vi "Main.vi"() -> ()   [LabVIEW 2019]
uses:
  controls/Data.ctl
  controls/UIRef.ctl
  controls/daqtypedef.ctl
  <vilib>/measure/NI_MABase.lvlib
panel:
  in  "Acquire":bool
  in  "Exit":bool
  out "Raw Data":waveform(dbl)(graph)
  out "Status Bar":string
  # "Laboratorium OSP"
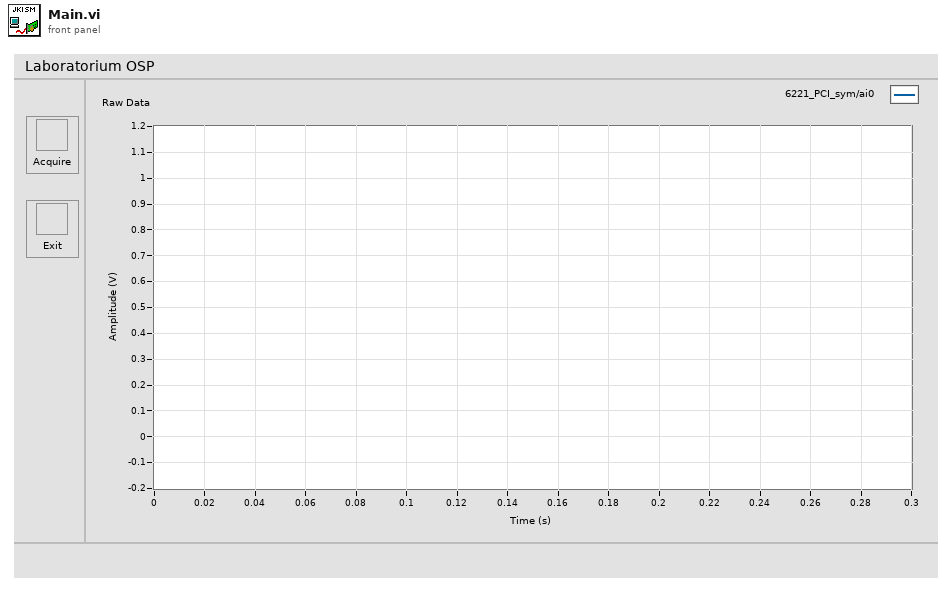
[diagram p1: front panel]
types:
  T1 = enum32{"Invalid", "Standard", "Closed", "Hidden", "Minimized", "Maximized"}
  T2 = enum32{"invalid app kind", "Development System", "Run Time System", "Student Edition", "Embedded LabVIEW", "Evaluation", "Custom"}
  T3 = typedef "Data.ctl" = cluster{"UICtlRef":T4, "DAQmxChannel":T5, "DAQmx Task Name":refnum<k21>, "Acquired Signal":waveform(dbl), "configuration file path":path, "taskout":refnum<k21>}
  T4 = typedef "UIRef.ctl" = cluster{"Acquire Btn":refnum<vi>, "Exit Btn":refnum<vi>, "Status":refnum<vi>, "WGraph":refnum<vi>}
  T5 = typedef "daqtypedef.ctl" = cluster{"PhysicalChanName":tag, "AI.Max":dbl, "AI.Min":dbl, "SampQuant.SampPerChan":dbl, "SampClk.Rate":dbl}
  T6 = cluster{"Core":cluster{"Current VI Reference":refnum<vi>, "Close Panel on Exit?":bool}, "Data":T3}
  T7 = cluster{"Current VI Reference":refnum<vi>, "Close Panel on Exit?":bool}
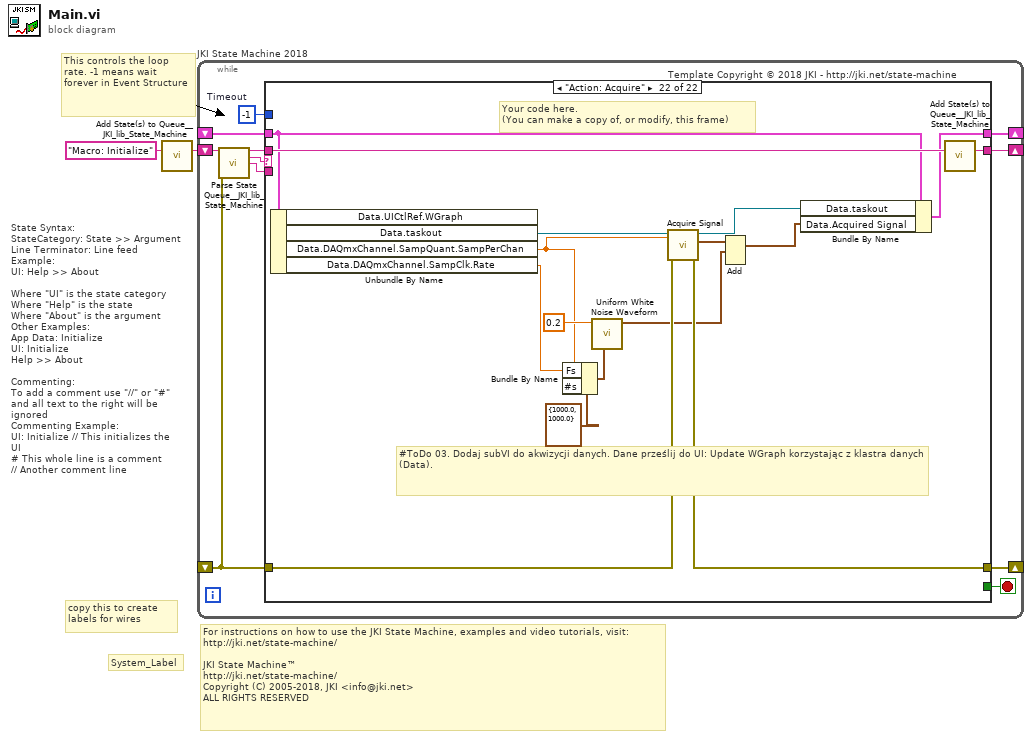
[diagram p0: block diagram]
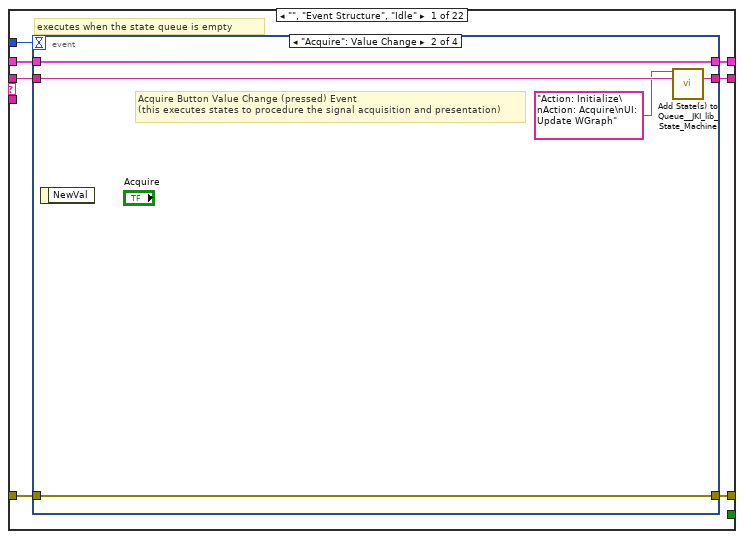
[diagram p2: hidden frame]
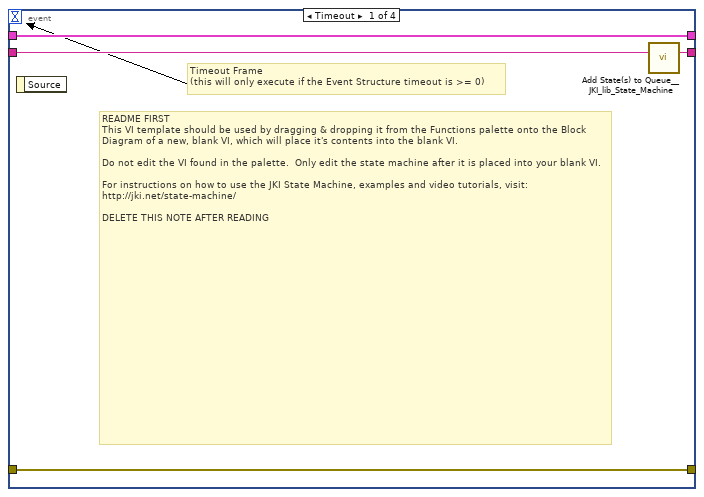
[diagram p3: hidden frame]
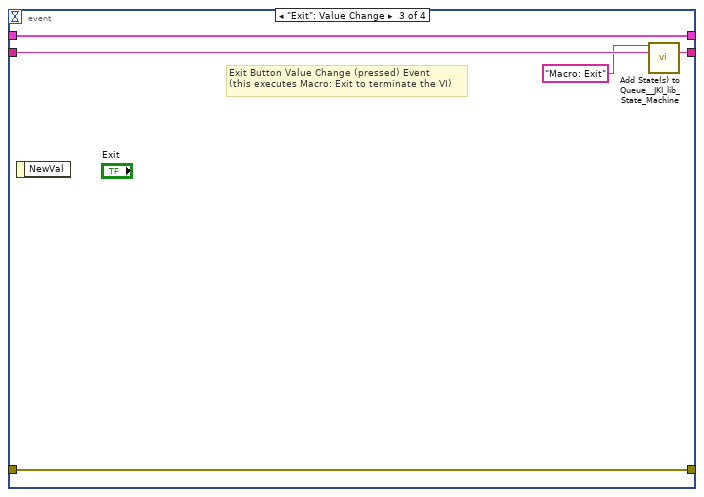
[diagram p4: hidden frame]
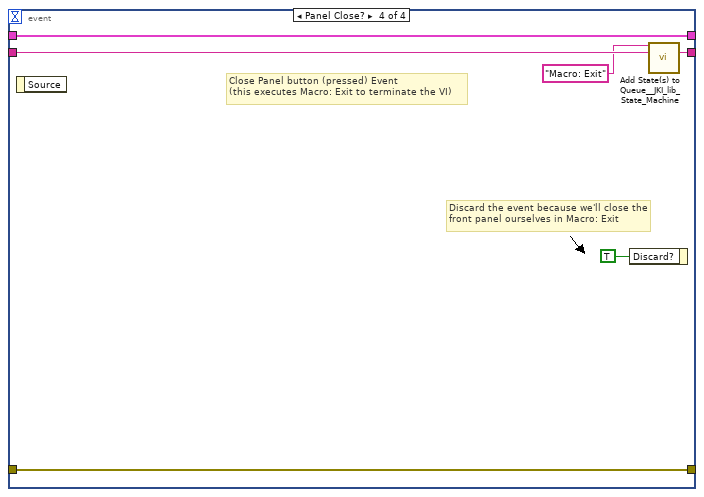
[diagram p5: hidden frame]
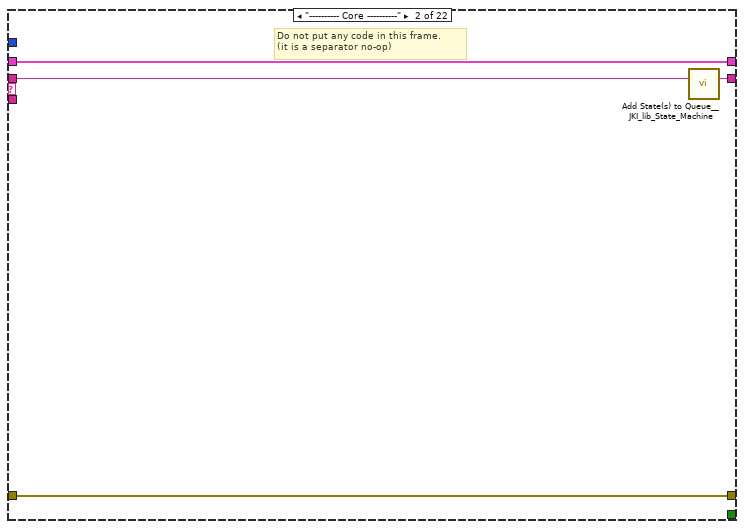
[diagram p6: hidden frame]
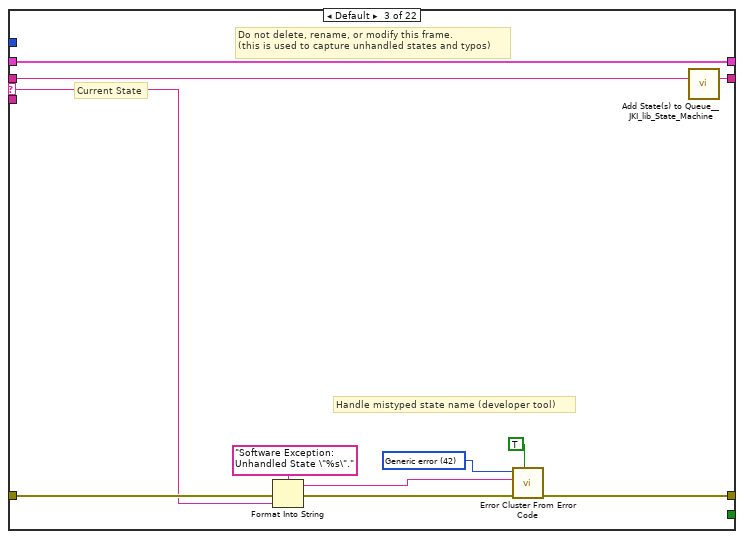
[diagram p7: hidden frame]
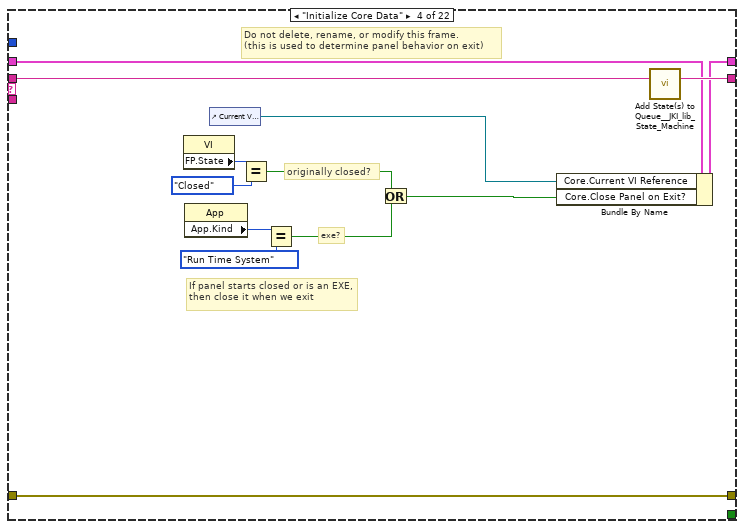
[diagram p8: hidden frame]
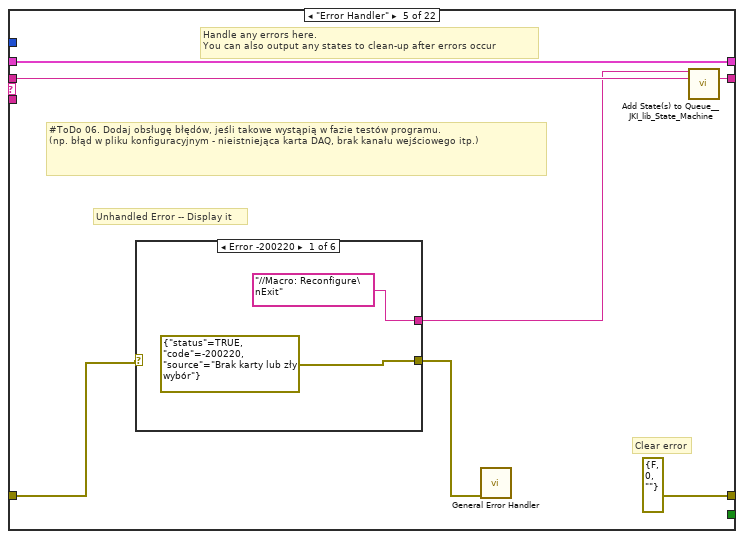
[diagram p9: hidden frame]
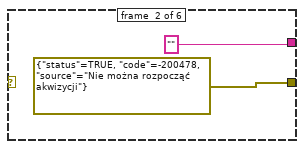
[diagram p10: hidden frame]
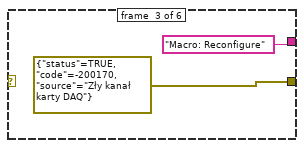
[diagram p11: hidden frame]
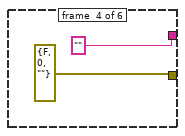
[diagram p12: hidden frame]
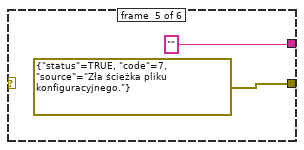
[diagram p13: hidden frame]
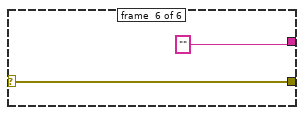
[diagram p14: hidden frame]
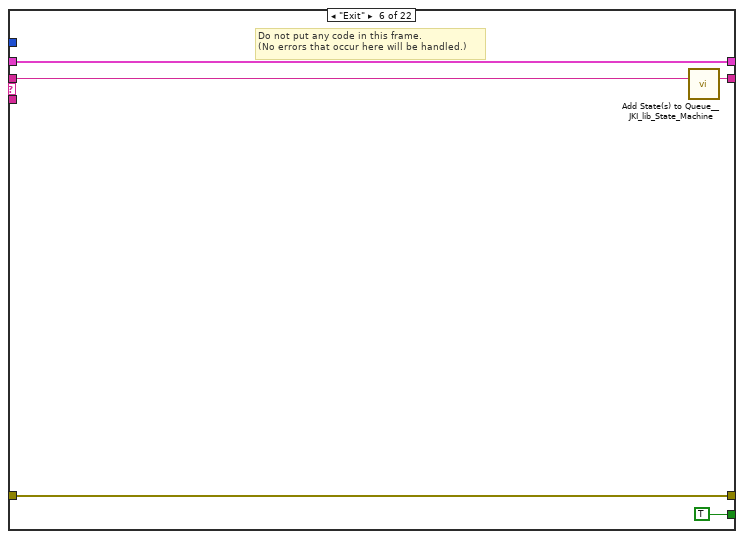
[diagram p15: hidden frame]
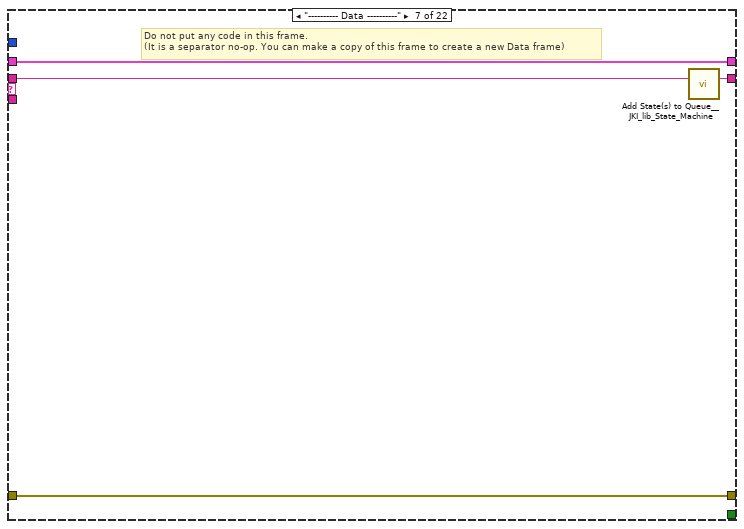
[diagram p16: hidden frame]
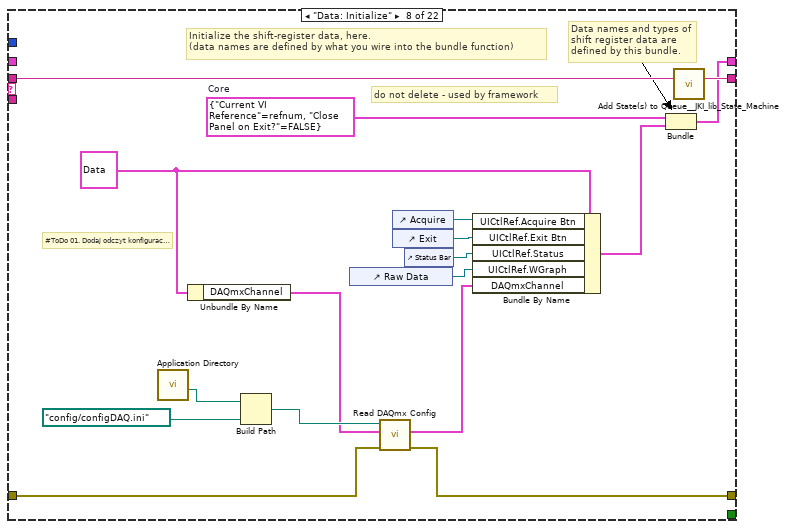
[diagram p17: hidden frame]
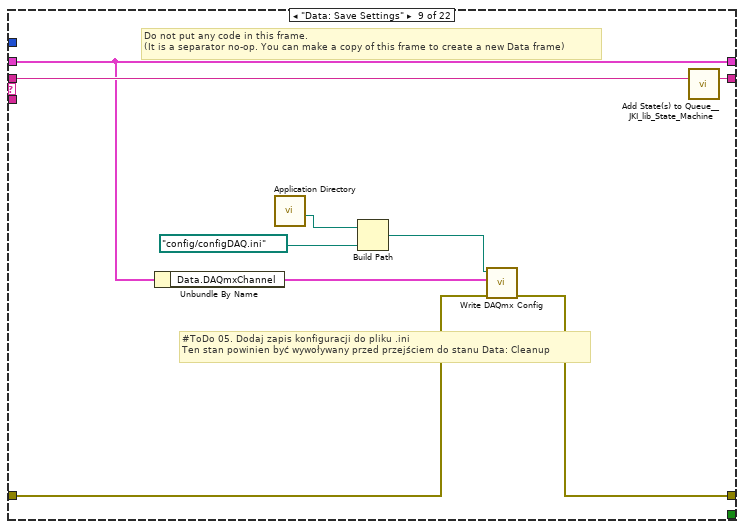
[diagram p18: hidden frame]
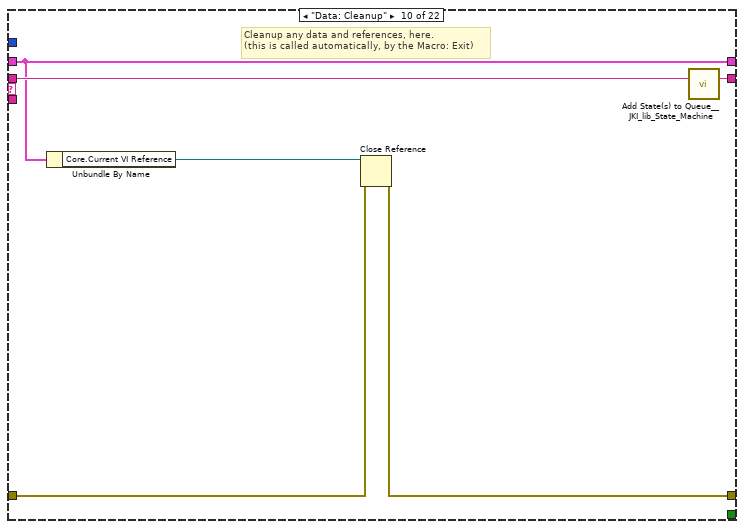
[diagram p19: hidden frame]
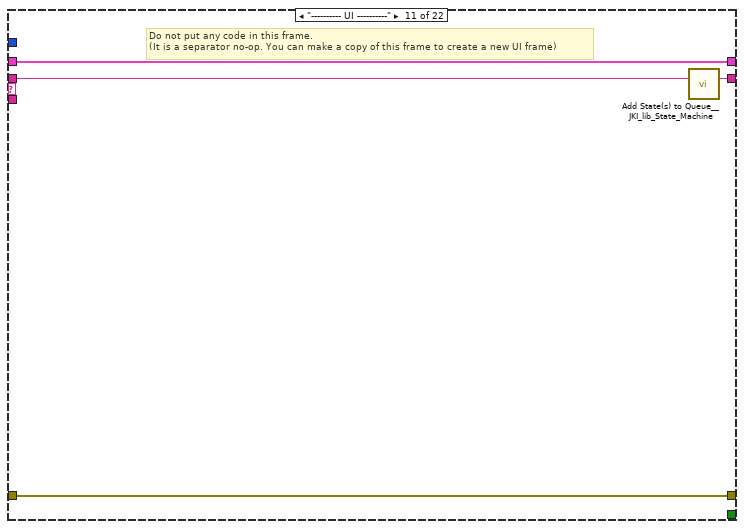
[diagram p20: hidden frame]
diagram:
  # "For instructions on how to use the JKI State Machine, examples and video tutorials, visit:\nhttp://jki.net/state-machine/\n\nJKI State Machine™\nhttp://jki.net/state-machine/\nCopyright (C) 2005-2018, JKI <info@jki.net>\nALL RIGHTS RESERVED"
  # "State Syntax:\nStateCategory: State >> Argument\nLine Terminator: Line feed\nExample:\nUI: Help >> About\n\nWhere \"UI\" is the state category\nWhere \"Help\" is the state\nWhere \"About\" is the argument\nOther Examples:\nApp Data: Initialize\nUI: Initialize\nHelp >> About\n\nCommenting:\nTo add a comment use \"//\" or \"#\" and all text to the right will be ignored\nCommenting Example:\nUI: Initialize // This initializes the UI\n# This whole line is a comment\n// Another comment line"
  # "copy this to create labels for wires"
  # "This controls the loop rate. -1 means wait forever in Event Structure"
  # "System_Label"
  n1 = call <vilib>:"Add State(s) to Queue__JKI_lib_State_Machine.vi"("State(s) in (\"\")"="Macro: Initialize") -> ("States Out"=w2:string)  [unwired: 14 in]
  n2 = while "JKI State Machine 2018" {
    shift-right: [w6] -> _
    shift-left: _ -> [w5]
    shift-right: [w9] -> _
    shift-left: _ -> [w3]
    shift-right: [w8] -> _
    shift-left: w2 -> [w10]
    stop <- w7 stop-if-true
    w4 = -1  # Timeout
    # "Template Copyright © 2018 JKI - http://jki.net/state-machine"
    n3 = call <vilib>:"Parse State Queue__JKI_lib_State_Machine.vi"("State Queue"=w10, "Error In (no error)"=w3) -> ("Remaining States"=w12:string, "Current State"=w13:string, "Arguments"=w11:string)  [unwired: 11 in]
    n4 = case shown="\"Action: Acquire\"" w13 {
      selector: w13 -> [_ _ w45 _ _ _ _ _ _ _ _ _ _ _ _ _ _ _ _ _ _ _]
      tunnel: w12 -> [w20 w44 w49 w68 w75 w92 w96 w113 w122 w128 w132 w137 w141 w147 w160 w229 w234 w240 w253 w257 w265 w281]
      tunnel: w11 -> [_ _ _ _ _ _ _ _ _ _ _ _ _ w142 w155 _ _ _ _ _ _ _]
      tunnel: w5 -> [w18 w41 w47 w61 w72 w90 w93 _ w120 w123 w129 w134 w139 w145 w157 w226 w231 w238 w250 w254 w260 w276]
      tunnel: [w17 w42 w51 w65 errorcluster {"status"=FALSE, "code"=0, "source"=""} ("error out") w89 w94 w103 w114 w124 w130 w135 w138 w143 w152 w227 w232 w236 w251 w255 w262 w277] -> w9
      tunnel: w3 -> [w16 w42 w50 w65 w70 w89 w94 w104 w115 w125 w130 w135 w138 w144 w158 w227 w232 w235 w251 w255 w263 w278]
      tunnel: [w19 w43 w48 w67 w74 w91 w95 w112 w121 w127 w131 w136 w140 w146 w159 w228 w233 w239 w252 w256 w264 w280] -> w8
      tunnel: [_ _ _ _ _ TRUE _ _ _ _ _ _ _ _ _ _ _ _ _ _ _ _] -> w7
      tunnel: [w15 w41 w47 w66 w72 w90 w93 w111 w120 w123 w129 w134 w139 w145 w157 w226 w231 w238 w250 w254 w259 w273] -> w6
      tunnel: w4 -> [w14 _ _ _ _ _ _ _ _ _ _ _ _ _ _ _ _ _ _ _ _ _]
      frame "", "Event Structure", "Idle" {
        # "executes when the state queue is empty"
        n5 = event shown="[1] \"Acquire\": Value Change" {
          selector: _ -> [_ _ _ _]
          dyn-events: _ -> [_ _ _ _]
          timeout: w14 -> [_ _ _ _]
          tunnel: w20 -> [w24 w29 w34 w40]
          tunnel: [w23 w28 w33 w39] -> w19
          tunnel: w18 -> [w21 w25 w31 w37]
          tunnel: [w22 w27 w32 w38] -> w17
          tunnel: w16 -> [w22 w27 w32 w38]
          tunnel: [w21 w25 w31 w37] -> w15
          event Timeout {
            # "README FIRST\nThis VI template should be used by dragging & dropping it from the Functions palette onto the Block Diagram of a new, blank VI, which will place it's contents into the blank VI.\n\nDo not edit the VI found in the palette.  Only edit the state machine after it is placed into your blank VI.\n\nFor instructions on how to use the JKI State Machine, examples and video tutorials, visit:\nhttp://jki.net/state-machine/\n\nDELETE THIS NOTE AFTER READING"
            # "Timeout Frame\n(this will only execute if the Event Structure timeout is >= 0)"
            n6 = event-data() -> ()  [unwired: 1 in, 1 out]
            n7 = call <vilib>:"Add State(s) to Queue__JKI_lib_State_Machine.vi"("State(s) in (\"\")"=w24) -> ("States Out"=w23:string)  [unwired: 14 in]
          }
          event "Acquire": Value Change {
            # "Acquire Button Value Change (pressed) Event\n(this executes states to procedure the signal acquisition and presentation)"
            n8 = event-data() -> ()  [unwired: 1 in, 1 out]
            n9 = call <vilib>:"Add State(s) to Queue__JKI_lib_State_Machine.vi"("State(s) in Front (\"\")"="Action: Initialize\nAction: Acquire\nUI: Update WGraph", "State(s) in (\"\")"=w29) -> ("States Out"=w28:string)  [unwired: 13 in]
          }
          event "Exit": Value Change {
            # "Exit Button Value Change (pressed) Event\n(this executes Macro: Exit to terminate the VI)"
            n10 = event-data() -> ()  [unwired: 1 in, 1 out]
            n11 = call <vilib>:"Add State(s) to Queue__JKI_lib_State_Machine.vi"("State(s) in Front (\"\")"="Macro: Exit", "State(s) in (\"\")"=w34) -> ("States Out"=w33:string)  [unwired: 13 in]
          }
          event Panel Close? {
            # "Discard the event because we'll close the front panel ourselves in Macro: Exit"
            # "Close Panel button (pressed) Event\n(this executes Macro: Exit to terminate the VI)"
            n12 = event-data() -> ()  [unwired: 1 in, 1 out]
            n13 = event-data("Discard?"=TRUE) -> ()  [unwired: 1 in, 1 out]
            n14 = call <vilib>:"Add State(s) to Queue__JKI_lib_State_Machine.vi"("State(s) in Front (\"\")"="Macro: Exit", "State(s) in (\"\")"=w40) -> ("States Out"=w39:string)  [unwired: 13 in]
          }
        }
      }
      frame "---------- Core ----------" {
        # "Do not put any code in this frame.\n(it is a separator no-op)"
        n15 = call <vilib>:"Add State(s) to Queue__JKI_lib_State_Machine.vi"("State(s) in (\"\")"=w44) -> ("States Out"=w43:string)  [unwired: 14 in]
      }
      frame Default {
        w54 = 42 items=["No error", "Argument error", "Memory is full", "Out of zone", "End of file", "File already open", "Generic file I/O error", "File not found", "File permission error", "Disk is full", "Duplicate path", "Too many files open", "System feature not enabled", "Resource file not found", "Cannot add resource", "Resource not found", "Image not found", "Image memory error", "Pen does not exist", "Config type invalid", "Config token not found", "Config parse error", "Config memory error", "Bad external code format", "Bad external code offset", "External code not present", "Null window", "Destroy window error", "Null menu", "Print aborted", "Bad print record", "Print driver error", "Windows error during printing", "Memory error during printing", "Print dialog error", "Generic print error", "Invalid device refnum", "Device not found", "Device parameter error", "Device unit error", "Cannot open device", "Device call aborted", "Generic error", "Cancelled by user", "Object ID too low", "Object ID too high", "Object not in heap", "Unknown heap", "Unknown object (invalid DefProc)", "Unknown object (DefProc not in table)", "Message out of range", "Invalid (null) method", "Unknown message", "Manager call not supported", "Bad address", "Network operation in progress", "Network operation timed out", "Connection is busy", "Network attribute not supported", "Network error", "Address in use", "System out of memory", "Connection aborted", "Connection refused", "Not connected", "Already connected", "Connection closed", "Initialization error (interapplication manager)", "Bad occurrence", "Wait on unbound occurrence handler", "Occurrence queue overflow", "Datalog type conflict", "Unused", "Unrecognized type (interapplication manager)", "Memory corrupt", "Failed to make temporary DLL", "Old CIN version", "Drag socket not found", "Failed to load drop-object", "Failed to register OLE object", "Failed to release OLE object", "Format specifier type mismatch", "Unknown format specifier", "Too few format specifiers", "Too many format specifiers", "Scan failed", "Newer CIN version", "Error converting to variant", "Runtime menu error", "Password tampered", "Variant attribute not found", "Incompatible variant data type", "Event data is not available", "Event Store is not present", "Occurrence is not found", "Event Queue is not created", "Event info is not available", "Refnum passed is NULL", "Error retrieving Class GUID", "Error retrieving CoClass GUID", "Error retrieving TypeLib GUID.", "Bad built application magic bytes.", "Specific driver is different from the specific driver associated with the Logical Name.", "There is no session opened to the class driver.", "Max Error", "MAX - Error with config objects", "MAX - Error loading configuration", "MAX - Group not supported"]
        # "Current State"
        # "Do not delete, rename, or modify this frame.\n(this is used to capture unhandled states and typos)"
        # "Handle mistyped state name (developer tool)"
        n16 = Format Into String(format string="Software Exception: Unhandled State \"%s\"." ("message"), error in=w50, w45) -> (resulting string=w53:string, error out=w52:errorcluster)  [unwired: 1 in]
        n17 = call <vilib>:"Error Cluster From Error Code.vi"("show call chain? (False)"=TRUE, "error in (no error)"=w52, "error message (\"\")"=w53, "error code (0)"=w54) -> ("error out"=w51:errorcluster)  [unwired: 5 in]
        n18 = call <vilib>:"Add State(s) to Queue__JKI_lib_State_Machine.vi"("State(s) in (\"\")"=w49) -> ("States Out"=w48:string)  [unwired: 14 in]
      }
      frame "Initialize Core Data" {
        # "Do not delete, rename, or modify this frame.\n(this is used to determine panel behavior on exit)"
        # "originally closed?"
        # "exe?"
        # "If panel starts closed or is an EXE, then close it when we exit"
        n19 = property class="VI"() -> ("FP.State"=w58:T1)  [unwired: 2 in, 2 out]
        n20 = property class="App"() -> ("App.Kind"=w64:T2)  [unwired: 2 in, 2 out]
        n21 = control-ref of="Current VI Reference"() -> (w59:refnum<vi>)
        n22 = Equal?(x=w58, y=T1."Closed" ("Front Panel Window:State")) -> (x = y?=w56:bool)
        n23 = Equal?(x=w64, y=T2."Run Time System" ("Application:Kind")) -> (x = y?=w62:bool)
        n24 = Or(x=w56, y=w62) -> (x .or. y?=w60:bool)
        n25 = Bundle By Name(cluster=w61, "Core.Current VI Reference"=w59, "Core.Close Panel on Exit?"=w60) -> (w66:T6)
        n26 = call <vilib>:"Add State(s) to Queue__JKI_lib_State_Machine.vi"("State(s) in (\"\")"=w68) -> ("States Out"=w67:string)  [unwired: 14 in]
      }
      frame "Error Handler" {
        # "#ToDo 06. Dodaj obsługę błędów, jeśli takowe wystąpią w fazie testów programu.\n(np. błąd w pliku konfiguracyjnym - nieistniejąca karta DAQ, brak kanału wejściowego itp.)"
        # "Unhandled Error -- Display it"
        # "Handle any errors here.\nYou can also output any states to clean-up after errors occur"
        # "Clear error"
        n27 = case shown="Error -200220" w70 {
          selector: w70 -> [_ _ _ _ _ w87]
          tunnel: [errorcluster {"status"=TRUE, "code"=-200220, "source"="Brak karty lub zły wybór"} ("error in (no error)") errorcluster {"status"=TRUE, "code"=-200478, "source"="Nie można rozpocząć akwizycji"} ("error in (no error)") errorcluster {"status"=TRUE, "code"=-200170, "source"="Zły kanał karty DAQ"} ("error in (no error)") errorcluster {"status"=FALSE, "code"=0, "source"=""} ("error in (no error)") errorcluster {"status"=TRUE, "code"=7, "source"="Zła ścieżka pliku konfiguracyjnego."} ("error in (no error)") w87] -> w71
          tunnel: ["//Macro: Reconfigure\nExit" "" "Macro: Reconfigure" "" "" ""] -> w69
          frame #0 {
          }
          frame #1 {
          }
          frame #2 {
          }
          frame #3 {
          }
          frame #4 {
          }
          frame #5 {
          }
        }
        n28 = call <vilib>:"General Error Handler.vi"("error in (no error)"=w71) -> ()  [unwired: 10 in, 5 out]
        n29 = call <vilib>:"Add State(s) to Queue__JKI_lib_State_Machine.vi"("State(s) in Front (\"\")"=w69, "State(s) in (\"\")"=w75) -> ("States Out"=w74:string)  [unwired: 13 in]
      }
      frame "Exit" {
        # "Do not put any code in this frame.\n(No errors that occur here will be handled.)"
        n30 = call <vilib>:"Add State(s) to Queue__JKI_lib_State_Machine.vi"("State(s) in (\"\")"=w92) -> ("States Out"=w91:string)  [unwired: 14 in]
      }
      frame "---------- Data ----------" {
        # "Do not put any code in this frame.\n(It is a separator no-op. You can make a copy of this frame to create a new Data frame)"
        n31 = call <vilib>:"Add State(s) to Queue__JKI_lib_State_Machine.vi"("State(s) in (\"\")"=w96) -> ("States Out"=w95:string)  [unwired: 14 in]
      }
      frame "Data: Initialize" {
        w98 = T3 {"UICtlRef"={"Acquire Btn"=refnum, "Exit Btn"=refnum, "Status"=refnum, "WGraph"=refnum}, "DAQmxChannel"={"PhysicalChanName"="", "AI.Max"=0.0, "AI.Min"=0.0, "SampQuant.SampPerChan"=0.0, "SampClk.Rate"=0.0}, "DAQmx Task Name"="", "Acquired Signal"={"t0"=timestamp(0 s since 1904-01-01), "dt"=0.0, "Y"=[]}, "configuration file path"=path "", "taskout"=""} ("Data")
        w110 = T7 {"Current VI Reference"=refnum, "Close Panel on Exit?"=FALSE}  # Core
        # "#ToDo 01. Dodaj odczyt konfiguracji akwizycji danych, z pliku."
        # "do not delete - used by framework"
        # "Data names and types of shift register data are defined by this bundle."
        # "Initialize the shift-register data, here.\n(data names are defined by what you wire into the bundle function)"
        n32 = call <vilib>:"Application Directory.vi"() -> ("Application Directory"=w101:path)
        n33 = Unbundle By Name(w98) -> ("DAQmxChannel"=w97:T5)
        n34 = Build Path(base path=w101, name or relative path=path "config/configDAQ.ini" ("configuration file path")) -> (appended path=w99:path)
        n35 = control-ref of="Raw Data"() -> (w106:refnum<vi>)
        n36 = call "Read DAQmx Config.vi"("error in (no error)"=w104, "DAQmxChannel"=w97, "configuration file path"=w99) -> ("error out"=w103:errorcluster, "DAQmx Channel out"=w102:T5)  [unwired: 6 in, 1 out]
        n37 = control-ref of="Acquire"() -> (w109:refnum<vi>)
        n38 = control-ref of="Exit"() -> (w108:refnum<vi>)
        n39 = control-ref of="Status Bar"() -> (w107:refnum<vi>)
        n40 = Bundle By Name(cluster=w98, "UICtlRef.Acquire Btn"=w109, "UICtlRef.Exit Btn"=w108, "UICtlRef.Status"=w107, "UICtlRef.WGraph"=w106, "DAQmxChannel"=w102) -> (w105:T3)
        n41 = Bundle("Core"=w110, "Data"=w105) -> (w111:T6)  [unwired: 1 in]
        n42 = call <vilib>:"Add State(s) to Queue__JKI_lib_State_Machine.vi"("State(s) in (\"\")"=w113) -> ("States Out"=w112:string)  [unwired: 14 in]
      }
      frame "Data: Save Settings" {
        # "#ToDo 05. Dodaj zapis konfiguracji do pliku .ini\nTen stan powinien być wywoływany przed przejściem do stanu Data: Cleanup"
        # "Do not put any code in this frame.\n(It is a separator no-op. You can make a copy of this frame to create a new Data frame)"
        n43 = Unbundle By Name(w120) -> ("Data.DAQmxChannel"=w119:T5)
        n44 = call <vilib>:"Application Directory.vi"() -> ("Application Directory"=w118:path)
        n45 = Build Path(base path=w118, name or relative path=path "config/configDAQ.ini" ("configuration file path")) -> (appended path=w116:path)
        n46 = call "Write DAQmx Config.vi"("error in (no error)"=w115, "DAQmxChannel"=w119, "configuration file path"=w116) -> ("error out"=w114:errorcluster)  [unwired: 8 in]
        n47 = call <vilib>:"Add State(s) to Queue__JKI_lib_State_Machine.vi"("State(s) in (\"\")"=w122) -> ("States Out"=w121:string)  [unwired: 14 in]
      }
      frame "Data: Cleanup" {
        # "Cleanup any data and references, here.\n(this is called automatically, by the Macro: Exit)"
        n48 = Unbundle By Name(w123) -> ("Core.Current VI Reference"=w126:refnum<vi>)
        n49 = Close Reference(reference=w126, error in (no error)=w125) -> (error out=w124:errorcluster)
        n50 = call <vilib>:"Add State(s) to Queue__JKI_lib_State_Machine.vi"("State(s) in (\"\")"=w128) -> ("States Out"=w127:string)  [unwired: 14 in]
      }
      frame "---------- UI ----------" {
        # "Do not put any code in this frame.\n(It is a separator no-op. You can make a copy of this frame to create a new UI frame)"
        n51 = call <vilib>:"Add State(s) to Queue__JKI_lib_State_Machine.vi"("State(s) in (\"\")"=w132) -> ("States Out"=w131:string)  [unwired: 14 in]
      }
      frame "UI: Update WGraph" {
        # "#ToDo 04. Dodaj wykreślanie zarejestrowanych danych, na wykresie."
        # "Do not put any code in this frame.\n(It is a separator no-op. You can make a copy of this frame to create a new UI frame)"
        n52 = Unbundle By Name(w134) -> ("Data.Acquired Signal"=w133:waveform(dbl))
        "Raw Data" <- w133
        n53 = shared-variable ".\\Untitled Library 1.lvlib\\Waveform"(w133) -> ()  [unwired: 1 in, 1 out]
        n54 = call "czujka.vi"("waveform in"=w133) -> ()  [unwired: 9 in, 2 out]
        n55 = call <vilib>:"Add State(s) to Queue__JKI_lib_State_Machine.vi"("State(s) in (\"\")"=w137) -> ("States Out"=w136:string)  [unwired: 14 in]
      }
      frame "UI: Initialize" {
        # "Initialize the User Interface, here.\n(this is called automatically, by the Macro: Init)"
        n56 = call <vilib>:"Add State(s) to Queue__JKI_lib_State_Machine.vi"("State(s) in (\"\")"=w141) -> ("States Out"=w140:string)  [unwired: 14 in]
      }
      frame "UI: Cursor Set" {
        # "Argument"
        # "Set and Unset Cursor Busy.\n(Usage: \"UI: Cursor Set >> Busy|Idle\")"
        n57 = case shown="\"Idle\", Default" w142 {
          tunnel: w144 -> [w149 w151]
          tunnel: [w148 w150] -> w143
          frame "Idle", Default {
            n58 = call <vilib>:"Unset Busy.vi"("error in (no error)"=w149) -> ("error out"=w148:errorcluster)  [unwired: 10 in]
          }
          frame "Busy" {
            n59 = call <vilib>:"Set Busy.vi"("error in (no error)"=w151) -> ("error out"=w150:errorcluster)  [unwired: 9 in, 1 out]
          }
        }
        n60 = call <vilib>:"Add State(s) to Queue__JKI_lib_State_Machine.vi"("State(s) in (\"\")"=w147) -> ("States Out"=w146:string)  [unwired: 14 in]
      }
      frame "UI: Front Panel State" {
        # "Argument"
        # "Set Front Panel Open or Closed\n(Usage: \"UI: Front Panel State >> Open|Close\")"
        n61 = Unbundle By Name(w157) -> ("Core.Current VI Reference"=w156:refnum<vi>)
        n62 = case shown="\"Open\", \"Standard\", Default" w155 {
          tunnel: w158 -> [w166 w181 w192 w205 w218]
          tunnel: [w168 w182 w194 w207 w220] -> w153
          tunnel: w156 -> [w167 w179 w193 w206 w219]
          frame "Open", "Standard", Default {
            w161 = T1."Standard" ("State")
            n63 = property class="VI"(reference=w167, error in=w166) -> (reference out=w164:refnum<vi>, error out=w165:errorcluster, "FP.State"=w163:T1)
            n64 = Not Equal?(x=w163, y=w161) -> (x != y?=w162:bool)
            n65 = case shown="False" w162 {
              tunnel: [w172 w174] -> w168
              tunnel: w165 -> [w171 w174]
              tunnel: w164 -> [w170 _]
              tunnel: w161 -> [w169 _]
              frame True {
                n66 = invoke class="VI" method="FP.Open"(reference=w170, error in=w171, "Activate"=TRUE, "State"=w169) -> (error out=w172:errorcluster)  [unwired: 1 in, 4 out]
              }
              frame False {
              }
            }
          }
          frame "Close", "Closed" {
            n67 = property class="VI"(reference=w179, error in=w181) -> (reference out=w178:refnum<vi>, error out=w180:errorcluster, "FP.State"=w176:T1)
            n68 = Not Equal?(x=w176, y=T1."Closed" ("Front Panel Window:State")) -> (x != y?=w175:bool)
            n69 = case shown="True" w175 {
              tunnel: [w183 w186] -> w182
              tunnel: w180 -> [w183 w185]
              tunnel: w178 -> [_ w184]
              frame False {
              }
              frame True {
                n70 = invoke class="VI" method="FP.Close"(reference=w184, error in=w185) -> (error out=w186:errorcluster)  [unwired: 1 in, 2 out]
              }
            }
          }
          frame "Hidden", "Hide" {
            w187 = T1."Hidden" ("State")
            n71 = property class="VI"(reference=w193, error in=w192) -> (reference out=w190:refnum<vi>, error out=w191:errorcluster, "FP.State"=w189:T1)
            n72 = Not Equal?(x=w189, y=w187) -> (x != y?=w188:bool)
            n73 = case shown="True" w188 {
              tunnel: [w198 w199] -> w194
              tunnel: w191 -> [w197 w199]
              tunnel: w190 -> [w196 _]
              tunnel: w187 -> [w195 _]
              frame True {
                n74 = invoke class="VI" method="FP.Open"(reference=w196, error in=w197, "State"=w195) -> (error out=w198:errorcluster)  [unwired: 2 in, 4 out]
              }
              frame False {
              }
            }
          }
          frame "Minimize", "Minimized" {
            w200 = T1."Minimized" ("State")
            n75 = property class="VI"(reference=w206, error in=w205) -> (reference out=w203:refnum<vi>, error out=w204:errorcluster, "FP.State"=w202:T1)
            n76 = Not Equal?(x=w202, y=w200) -> (x != y?=w201:bool)
            n77 = case shown="True" w201 {
              tunnel: [w211 w212] -> w207
              tunnel: w204 -> [w210 w212]
              tunnel: w203 -> [w209 _]
              tunnel: w200 -> [w208 _]
              frame True {
                n78 = invoke class="VI" method="FP.Open"(reference=w209, error in=w210, "State"=w208) -> (error out=w211:errorcluster)  [unwired: 2 in, 4 out]
              }
              frame False {
              }
            }
          }
          frame "Maximize", "Maximized" {
            w213 = T1."Maximized" ("State")
            n79 = property class="VI"(reference=w219, error in=w218) -> (reference out=w216:refnum<vi>, error out=w217:errorcluster, "FP.State"=w215:T1)
            n80 = Not Equal?(x=w215, y=w213) -> (x != y?=w214:bool)
            n81 = case shown="True" w214 {
              tunnel: [w224 w225] -> w220
              tunnel: w217 -> [w223 w225]
              tunnel: w216 -> [w222 _]
              tunnel: w213 -> [w221 _]
              frame True {
                n82 = invoke class="VI" method="FP.Open"(reference=w222, error in=w223, "State"=w221) -> (error out=w224:errorcluster)  [unwired: 2 in, 4 out]
              }
              frame False {
              }
            }
          }
        }
        n83 = local write "Status Bar"("Ready for Acquisition" ("Status Bar")) -> ()
        n84 = call <vilib>:"Unset Busy.vi"("error in (no error)"=w153) -> ("error out"=w152:errorcluster)  [unwired: 10 in]
        n85 = call <vilib>:"Add State(s) to Queue__JKI_lib_State_Machine.vi"("State(s) in (\"\")"=w160) -> ("States Out"=w159:string)  [unwired: 14 in]
      }
      frame "---------- Macro ----------" {
        # "Do not put any code in this frame.\n(It is a separator no-op. You can make a copy of this frame to create a new Macro frame)"
        n86 = call <vilib>:"Add State(s) to Queue__JKI_lib_State_Machine.vi"("State(s) in (\"\")"=w229) -> ("States Out"=w228:string)  [unwired: 14 in]
      }
      frame "Macro: Reconfigure" {
        # "#Comment\nTen stan powoduje zapętlenie się w razie wystąpienia błedu. Zostaje tylko Kill!!!"
        # "Do not put any code in this frame.\n(It is a separator no-op. You can make a copy of this frame to create a new Macro frame)"
        n87 = call <vilib>:"Add State(s) to Queue__JKI_lib_State_Machine.vi"("State(s) in Front (\"\")"="Data: Initialize\nAction: Initialize", "State(s) in (\"\")"=w234) -> ("States Out"=w233:string)  [unwired: 13 in]
      }
      frame "Macro: Initialize" {
        w237 = "Data: Initialize\nInitialize Core Data\nUI: Initialize\nUI: Front Panel State >> Open"  # Data: Initialize Initialize Core Data UI: Initialize UI: Front Panel State >> Open
        # "Initialization Macro\n(This is called once, when the VI starts)"
        n88 = flat-sequence {
          frame #0 {
            "Status Bar" <- "Initializing Application: DAQ Configuration, Core Data, User Interface..." ("Status Bar")
          }
          frame #1 {
            n89 = Wait (ms)(milliseconds to wait=u32 2000) -> ()  [unwired: 1 out]
          }
        }
        n90 = call <vilib>:"Set Busy.vi"("error in (no error)"=w235) -> ("error out"=w236:errorcluster)  [unwired: 9 in, 1 out]
        n91 = call <vilib>:"Add State(s) to Queue__JKI_lib_State_Machine.vi"("State(s) in Front (\"\")"=w237, "State(s) in (\"\")"=w240) -> ("States Out"=w239:string)  [unwired: 13 in]
      }
      frame "Macro: Exit" {
        # "Exit Macro\n(This is called once, when the VI exits)"
        n92 = Unbundle By Name(w250) -> ("Core.Close Panel on Exit?"=w249:bool)
        n93 = local write "Status Bar"("Exitting application..." ("Status Bar")) -> ()
        n94 = Select(t="UI: Front Panel State >> Close", s=w249, f="") -> (s? t:f=w246:string)
        n95 = call <vilib>:"Add State(s) to Queue__JKI_lib_State_Machine.vi"("State(s) in (\"\")"=w246, "State(s) at Back (\"\")"="Data: Save Settings\nData: Cleanup\nExit") -> ("States Out"=w244:string)  [unwired: 13 in]
        n96 = call <vilib>:"Add State(s) to Queue__JKI_lib_State_Machine.vi"("State(s) in Front (\"\")"=w244, "State(s) in (\"\")"=w253) -> ("States Out"=w252:string)  [unwired: 13 in]
      }
      frame "---------- Action ----------" {
        # "Template Separator\n(You can make a copy of, or modify, this frame)"
        n97 = call <vilib>:"Add State(s) to Queue__JKI_lib_State_Machine.vi"("State(s) in (\"\")"=w257) -> ("States Out"=w256:string)  [unwired: 14 in]
      }
      frame "Action: Initialize" {
        # "#ToDo 02. Dodaj subVI do inicjalizacji akwizycji. Nie zapomnij dodać wyjścia \"task out\" do klastra danych (Data)."
        # "Your code here.\n(You can make a copy of, or modify, this frame)"
        n98 = Unbundle By Name(w260) -> ("Data.DAQmxChannel"=w261:T5)
        n99 = call "Initialize Acquisition.vi"("error in"=w263, "DAQmxChannel"=w261) -> ("error out"=w262:errorcluster, "task out"=w258:refnum<k21>)  [unwired: 8 in]
        n100 = Bundle By Name(cluster=w260, "Data.taskout"=w258) -> (w259:T6)
        n101 = call <vilib>:"Add State(s) to Queue__JKI_lib_State_Machine.vi"("State(s) in (\"\")"=w265) -> ("States Out"=w264:string)  [unwired: 14 in]
      }
      frame "Action: Acquire" {
        # "#ToDo 03. Dodaj subVI do akwizycji danych. Dane prześlij do UI: Update WGraph korzystając z klastra danych (Data)."
        # "Your code here.\n(You can make a copy of, or modify, this frame)"
        n102 = Unbundle By Name(w276) -> ("Data.taskout"=w279:refnum<k21>, "Data.DAQmxChannel.SampQuant.SampPerChan"=w270:dbl, "Data.DAQmxChannel.SampClk.Rate"=w266:dbl)  [unwired: 1 out]
        n103 = Bundle By Name(cluster=cluster{"Fs":dbl, "#s":dbl} {"Fs"=1000.0, "#s"=1000.0} ("sampling info"), "Fs"=w266, "#s"=w270) -> (w269:cluster{"Fs":dbl, "#s":dbl})
        n104 = call <vilib>:"Uniform White Noise Waveform.vi"("sampling info"=w269, "amplitude"=0.2) -> ("signal out"=w267:waveform(dbl))  [unwired: 8 in, 1 out]
        n105 = call "Acquire Signal.vi"("error in"=w278, "number of samples per channel"=w270, "task/channels in"=w279) -> ("error out"=w277:errorcluster, "data"=w274:waveform(dbl), "task out"=w275:refnum<k21>)  [unwired: 6 in]
        n106 = Add(1:w267, 2:w274) -> (0:w268:waveform(dbl))  [unwired: 1 in, 1 out]
        n107 = Bundle By Name(cluster=w276, "Data.taskout"=w275, "Data.Acquired Signal"=w268) -> (w273:T6)
        n108 = call <vilib>:"Add State(s) to Queue__JKI_lib_State_Machine.vi"("State(s) in (\"\")"=w281) -> ("States Out"=w280:string)  [unwired: 14 in]
      }
    }
  }
